vi "Add FullyCustom Profile RTM.vi"(8 "error in (no error)":errorcluster, 11 "Node Ptr":u64 format="%.0x") -> (0 "error out":errorcluster)   [LabVIEW 2011, in "Engine Sim System Explorer.lvlib"]
uses:
  Engine Sim System Explorer.lvlib
  TypeDefs/FullyCustomProfilesComp.ctl
  <vilib>/NI Veristand/Custom Device API/Custom Device Channel.ctl
  <vilib>/NI Veristand/Custom Device API/Custom Device Channel Type.ctl
  Shared/Engine Simulation Global.vi
  <vilib>/NI Veristand/Custom Device API/Get Item Property (Variant).vi
  <vilib>/NI Veristand/Custom Device API/Custom Device API.lvlib
  Engine Simulation Shared.lvlib
  <vilib>/NI Veristand/Custom Device Tools/Custom Device Utility Library/Custom Device Utility Library.lvlib
panel:
  in  "Tag":string
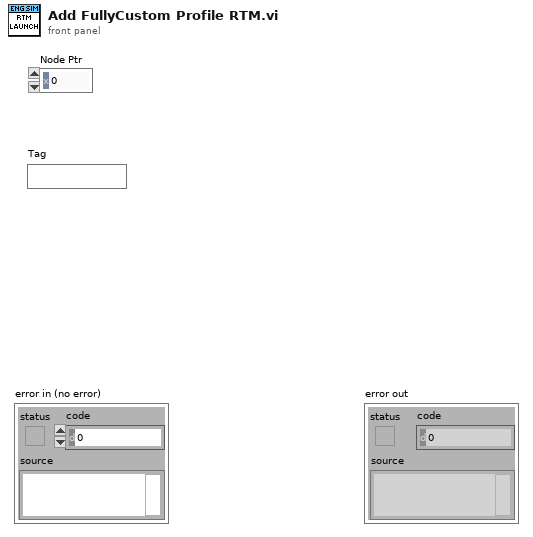
[diagram p1: front panel]
types:
  T1 = typedef "Custom Device API.lvlib/Custom Device Channel.ctl" = cluster{"Type":T2, "Units":string, "Default Value":dbl, "Faultable":bool, "Scalable":bool}
  T2 = typedef "Custom Device API.lvlib/Custom Device Channel Type.ctl" = enum16{"Input", "Output"}
  T3 = typedef "Engine Sim System Explorer.lvlib/FullyCustomProfilesComp.ctl" = cluster{"Name":string, "Offset?":bool}
  T4 = typedef "Custom Device API.lvlib/Custom Device Item Ref.ctl" = u64
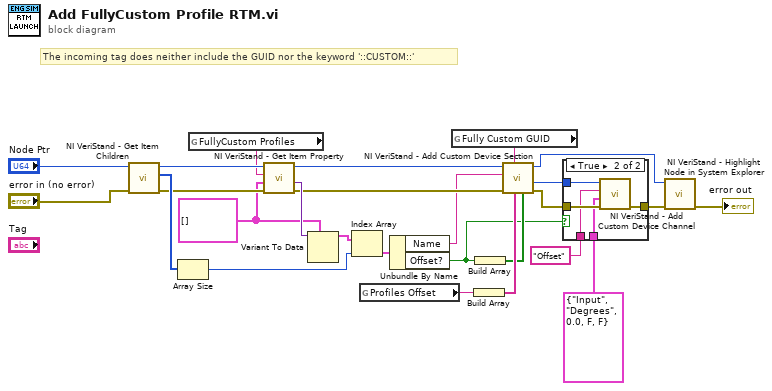
[diagram p0: block diagram]
diagram:
  w22 = T3[] []
  # "The incoming tag does neither include the GUID nor the keyword '::CUSTOM::'"
  n1 = call <vilib>:"NI VeriStand - Get Item Children.vi"("error in (no error)"="error in (no error)", "Item Ref in"="Node Ptr") -> ("error out"=w23:errorcluster, "Child Refs"=w26:T4[], "Item Ref out"=w24:T4)  [unwired: 6 in, 1 out]
  n2 = Array Size(array=w26) -> (size(s)=w18:i32)
  n3 = global read "Engine Simulation Global.vi" "FullyCustom Profiles"() -> (w3:string)
  n4 = call-poly <vilib>:"NI VeriStand - Get Item Property.vi"("error in (no error)"=w23, "Default Value"=w22, "Property Name"=w3, "Item Ref in"=w24) -> ("error out"=w16:errorcluster, "Value"=w25:variant, "Item Ref out"=w15:T4)  [unwired: 4 in, 1 out]
  n5 = Variant To Data(type=w22, Variant=w25) -> (data=w19:T3[])  [unwired: 1 in, 1 out]
  n6 = Index Array(array=w19, index=w18) -> (element=w17:T3)
  n7 = global read "Engine Simulation Global.vi" "Profiles Offset"() -> (w2:string)
  n8 = Unbundle By Name(w17) -> ("Name"=w14:string, "Offset?"=w7:bool)
  n9 = global read "Engine Simulation Global.vi" "Fully Custom GUID"() -> (w13:string)
  n10 = Build Array(w2) -> (w10:string[])
  n11 = Build Array(w7) -> (w9:bool[])
  n12 = call <vilib>:"NI VeriStand - Add Custom Device Section.vi"("Property Values"=w9, "Property names"=w10, "GUID (Default Section)"=w13, "error in (no error)"=w16, "Section Name"=w14, "Parent Ref in"=w15) -> ("error out"=w11:errorcluster, "Section Ptr"=w12:T4, "Parent Ref out"=w4:T4)  [unwired: 2 in, 1 out]
  n13 = case shown="True" w7 {
    tunnel: w12 -> [_ w32]
    tunnel: w11 -> [w27 w31]
    tunnel: [w27 w30] -> w6
    tunnel: "Offset" ("Profiles Offset") -> [_ w29]
    tunnel: T1 {"Type"=enum."Input", "Units"="Degrees", "Default Value"=0.0, "Faultable"=FALSE, "Scalable"=FALSE} ("Channel") -> [_ w28]
    frame False {
    }
    frame True {
      n14 = call <vilib>:"NI VeriStand - Add Custom Device Channel.vi"("error in (no error)"=w31, "Channel"=w28, "Channel Name"=w29, "Parent Ref in"=w32) -> ("error out"=w30:errorcluster)  [unwired: 4 in, 3 out]
    }
  }
  n15 = call <vilib>:"NI VeriStand - Highlight Node in System Explorer.vi"("error in (no error)"=w6, "Item Ref in"=w4) -> ("error out"=→"error out":errorcluster)  [unwired: 8 in, 1 out]
